vi "json manda.vi"() -> ()   [LabVIEW 2025]
uses:
  <vilib>/httpClient/PUTBuffer.vi
  <vilib>/httpClient/LabVIEWHTTPClient.lvlib
panel:
  out "headers":string
  out "body":string
  out "error out":errorcluster
  in  "stop":bool
  in  "Accionamiento":dbl
  in  "Rele":bool
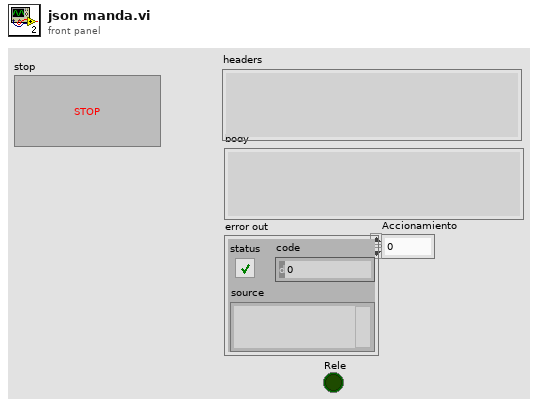
[diagram p1: front panel]
types:
  T1 = cluster{"Accionamiento":dbl, "Fecha":string, "Hora":string, "Rele":bool}
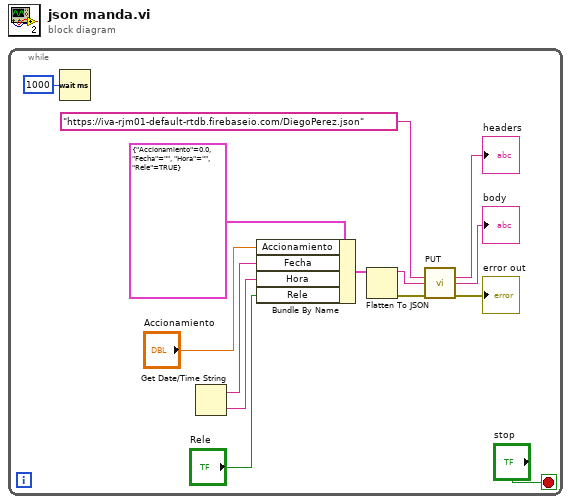
[diagram p0: block diagram]
diagram:
  n1 = while {
    stop <- "stop" stop-if-true
    n2 = Wait (ms)(milliseconds to wait=u32 1000) -> ()  [unwired: 1 out]
    n3 = Get Date/Time String() -> (date string=w2:string, time string=w1:string)  [unwired: 3 in]
    n4 = Bundle By Name(cluster=T1 {"Accionamiento"=0.0, "Fecha"="", "Hora"="", "Rele"=TRUE}, "Accionamiento"="Accionamiento", "Fecha"=w2, "Hora"=w1, "Rele"="Rele") -> (w8:T1)
    n5 = Flatten To JSON(anything=w8) -> (JSON string=w7:string, 11:w6:errorcluster)  [unwired: 2 in]
    n6 = call-poly <vilib>:"PUT.vi"("url"="https://iva-rjm01-default-rtdb.firebaseio.com/DiegoPerez.json", "buffer"=w7, "error in (no error)"=w6) -> ("headers"=→"headers":string, "body"=→"body":string, "error out"=→"error out":errorcluster)  [unwired: 9 in, 1 out]
  }
